vi "initMultiple.vi"(8 "错误输入（无错误）":errorcluster caption="errorIn", 10 "name":string[](array[string]), 11 "size(-1)":i32) -> (0 "错误输出":errorcluster caption="errorOut", 3 "refer":refnum<queue>[](array[refnum]))   [LabVIEW 2017]
uses:
  models/EMSGData.ctl
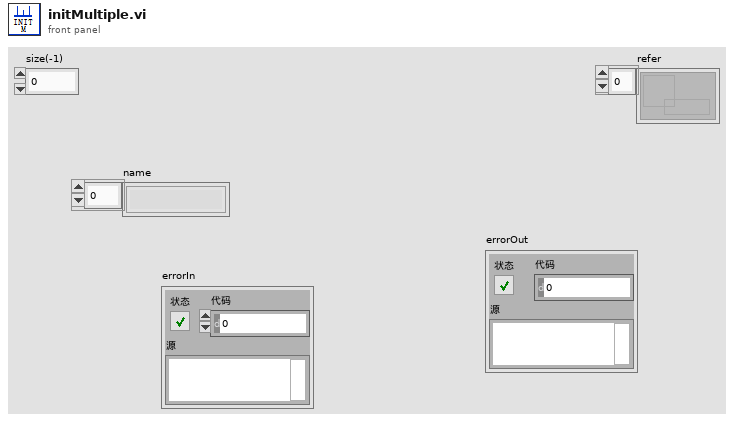
[diagram p1: front panel]
types:
  T1 = typedef "EMSGData.ctl" = cluster{"to":string, "from":string, "data":variant, "remark1":string, "remark 2":string}
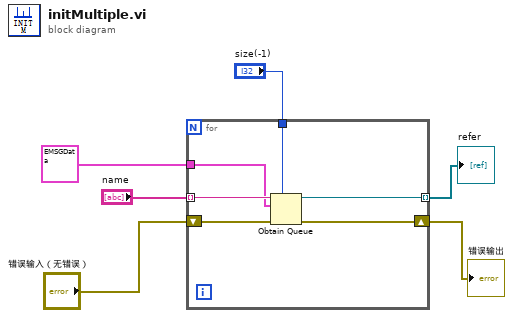
[diagram p0: block diagram]
diagram:
  n1 = for {
    tunnel: "name" -> [w12] mode=indexing
    tunnel: T1 {"to"="", "from"="", "data"=variant, "remark1"="", "remark 2"=""} ("EMSGData") -> [w11]
    shift-right: [w9] -> w3
    shift-left: "错误输入（无错误）" -> [w10]
    tunnel: [w8] -> w2 mode=indexing
    tunnel: "size(-1)" -> [w7]
    n2 = Obtain Queue(max queue size (-1, unlimited)=w7, name (unnamed)=w12, element data type=w11, error in (no error)=w10) -> (queue out=w8:refnum<queue>, error out=w9:errorcluster)  [unwired: 1 in, 1 out]
  }
  "错误输出" <- w3
  "refer" <- w2
